vi "Move From Output to Export Dir.vi"(0 "NI Build Specification in":refnum<class "Installer_LV.lvclass">, 11 "error IO":errorcluster) -> (4 "NI Build Specification out":refnum<class "Installer_LV.lvclass">, 15 "error out":errorcluster)   [LabVIEW 2017, in "CL_G3_VIComponentBuilder.lvlib" / "Installer_LV.lvclass"]
doc: "Moves the installer files from the Installer Output (specified in the build spec) to a new directory in the Component's Export directory. The new directory is named after the build spec name."
uses:
  Installer_LV.lvclass
  C:/Tool Chain Support/Software Module Builder/Source/Exports/Exports/Export.lvclass
  C:/Tool Chain Support/Software Module Builder/Source/Exports/NI Build Specification_LV/NI Build Specification_LV.lvclass
  Exports/Export.lvclass/Export.ctl
  NI Build Specification_LV/NI Build Specification_LV.lvclass/NI Build Specification_LV.ctl
  Exports/Accessors/Read Exported Build Specification Path.vi
  Exports/Accessors/Read Component Export Dir.vi
  NI Build Specification_LV/Accessors/Read Export's Build Spec Name.vi
  Exports/Accessors/Write Built Export's Full Path.vi
  <vilib>/xml/Load XML File.vi
  <vilib>/xml/Close Reference(Node).vi
  <vilib>/Utility/file.llb/Is Path and Not Empty.vi
  <vilib>/Utility/error.llb/Error Cluster From Error Code.vi
  NI Build Specification_LV/NI Build Specification_LV.lvclass
  <vilib>/xml/NI_XML.lvlib
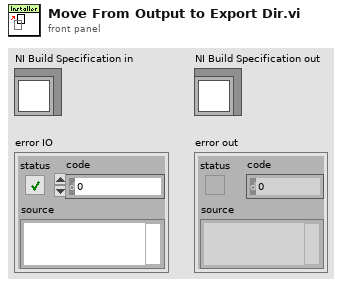
[diagram p1: front panel]
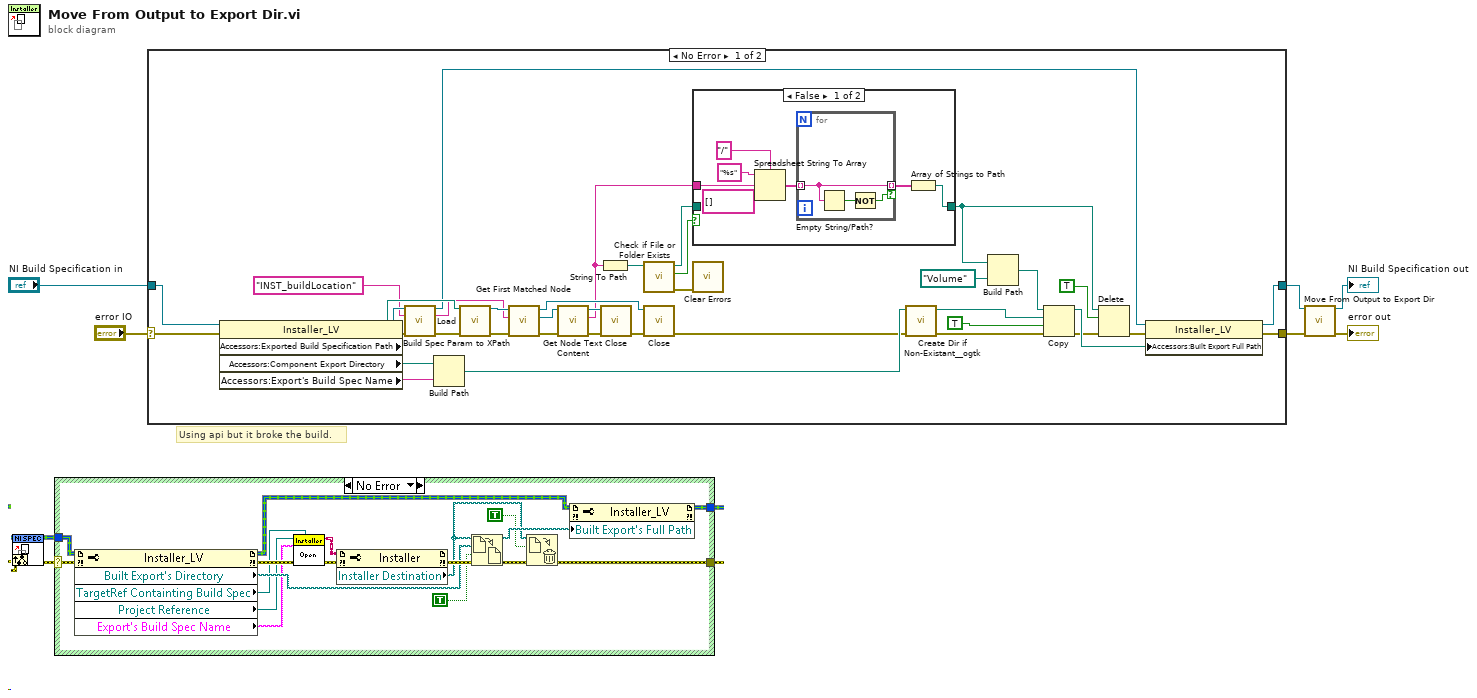
[diagram p0: block diagram]
diagram:
  # "Using api but it broke the build."
  n1 = case shown="No Error" "error IO" {
    selector: "error IO" -> [w25 w56]
    tunnel: [w44 w57] -> w2
    tunnel: "NI Build Specification in" -> [w26 w57]
    tunnel: [w22 w56] -> w5
    frame No Error {
      n2 = property class="Installer_LV"(reference=w26, error in=w25) -> (reference out=w21:refnum<class "Installer_LV.lvclass">, error out=w17:errorcluster, "Accessors:Exported Build Specification Path"=w35:path, "Accessors:Component Export Directory"=w7:path, "Accessors:Export's Build Spec Name"=w13:string)
      n3 = call-dynamic "Build Spec Param to XPath.vi"("NI Build Specification"=w21, "Build Spec Parameter Name"="INST_buildLocation", "error in (no error)"=w17) -> ("NI Build Specification"=w18:refnum<class "Installer_LV.lvclass">, "XPath to the specific build Spec Property"=w19:string, "error out"=w16:errorcluster)  [unwired: 10 in]
      n4 = Build Path(base path=w7, name or relative path=w13) -> (appended path=w11:path)
      n5 = call-poly <vilib>:"Load.vi"("path to XML document"=w35, "error in (no error)"=w16) -> ("DOM document out"=w37:refnum<k20>, "error out"=w36:errorcluster)  [unwired: 11 in, 1 out]
      n6 = call <vilib>:"Get First Matched Node.vi"("error in (no error)"=w36, "XPath expression"=w19, "node in"=w37) -> ("error out"=w39:errorcluster, "node result"=w40:refnum<k20>, "node out"=w38:refnum<k20>)  [unwired: 6 in]
      n7 = call <vilib>:"Get Node Text Content.vi"("error in (no error)"=w39, "node in"=w40) -> ("error out"=w33:errorcluster, "node text"=w27:string, "node out"=w34:refnum<k20>)  [unwired: 7 in]
      n8 = String To Path(string=w27) -> (path=w31:path)
      n9 = call-poly <vilib>:"Close.vi"("error in (no error)"=w33, "node"=w34) -> ("error out"=w32:errorcluster)  [unwired: 7 in]
      n10 = call <vilib>:"Check if File or Folder Exists.vi"("path"=w31) -> ("error out"=w28:errorcluster, "file or folder exists?"=w30:bool, "dup path"=w29:path)  [unwired: 8 in]
      n11 = call-poly <vilib>:"Close.vi"("error in (no error)"=w32, "node"=w38) -> ("error out"=w10:errorcluster)  [unwired: 7 in]
      n12 = case shown="False" w30 {
        tunnel: [w46 w55] -> w15
        tunnel: w27 -> [w45 _]
        tunnel: w29 -> [_ w55]
        frame False {
          n13 = Spreadsheet String To Array(delimiter (Tab)="/", format string="%s", spreadsheet string=w45, array type (2D Dbl)=string[] []) -> (array=w50:string[])
          n14 = for {
            tunnel: w50 -> [w53] mode=indexing
            tunnel: [w53] -> w51 mode=indexing if=w52
            n15 = Empty String/Path?(string/path=w53) -> (empty?=w54:bool)
            n16 = Not(x=w54) -> (.not. x?=w52:bool)
          }
          n17 = Array of Strings to Path(0:w51) -> (2:w46:path)  [unwired: 1 in]
        }
        frame True {
        }
      }
      n18 = call <vilib>:"Clear Errors.vi"("error in (no error)"=w28) -> ()  [unwired: 5 in, 2 out]
      n19 = call <userlib>:"Create Dir if Non-Existant__ogtk.vi"("error in (no error)"=w10, "Directory Path"=w11) -> ("error out"=w8:errorcluster, "dup Directory Path"=w9:path)  [unwired: 7 in, 1 out]
      n20 = Build Path(base path=w15, name or relative path=path "Volume") -> (appended path=w14:path)
      n21 = Copy(8:w8, 9:TRUE ("overwrite (F)"), 10:w9, 11:w14) -> (0:w24:errorcluster, 3:w41:path)  [unwired: 1 in, 1 out]
      n22 = Delete(path (use dialog)=w15, entire hierarchy (F)=TRUE, error in=w24) -> (error out=w23:errorcluster)  [unwired: 2 in, 2 out]
      n23 = property class="Installer_LV"(reference=w18, error in=w23, "Accessors:Built Export Full Path"=w41) -> (reference out=w44:refnum<class "Installer_LV.lvclass">, error out=w22:errorcluster)
    }
    frame Error {
    }
  }
  n24 = call-parent "Move From Output to Export Dir.vi"("NI Build Specification in"=w2, "error IO"=w5) -> ("NI Build Specification out"=→"NI Build Specification out":refnum<class "Installer_LV.lvclass">, "error out"=→"error out":errorcluster)  [unwired: 12 in]
